vi "ap1 (hw3).vi"() -> ()   [LabVIEW 2017]
panel:
  in  "STOP Button":bool
  out "Loop Iteration":dbl
  in  "Input (N)":dbl=1.0 min=1.0
  # "Problem AP1 (HW 3)"
  # "Input N has to be greater than 0"
  # "Patrik Sokolowski"
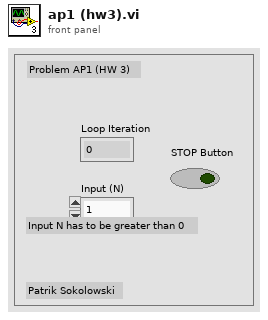
[diagram p1: front panel]
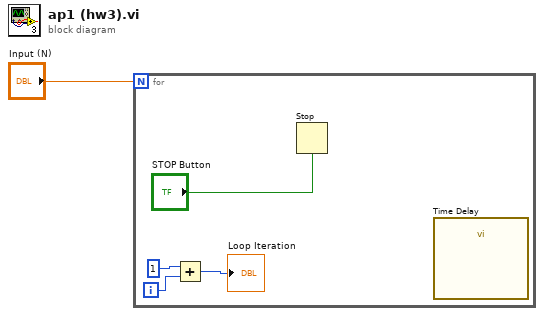
[diagram p0: block diagram]
diagram:
  n1 = for {
    N: "Input (N)" -> [_]
    i -> [w5]
    n2 = Add(x=1, y=w5) -> (x+y=→"Loop Iteration":i32)
    n3 = Stop(stop? (T)="STOP Button") -> ()
    n4 = call "Time Delay"() -> ()  [unwired: 11 in, 1 out]
  }
